vi "dcaccelerometer.vi"   [LabVIEW 2016]
uses:
  Scratch/FPGADCAccelerometer/DataTypes/DCAccelerometerSettings.ctl
  <vilib>/rvi/Emulation/niFpgaGetClockAttributes.vi
  <vilib>/rvi/Emulation/niFpgaSctlEmulationGetInTimedLoop.vi
  <vilib>/rvi/Emulation/niFpgaEmulationReportErrorSimple.vi
  <vilib>/rvi/Emulation/niFpgaEmulationIsFPGAContextNoSignature.vi
  <vilib>/rvi/errors/niFpgaSetErrorForExecOnDevCompSimple.vi
  <vilib>/rvi/eio/common/nirviEmuReportErrorAndStop.vi
  <vilib>/rvi/DataTransferAndStorage/Container/Common/niFpgaContainerGetUniqueNameForEmu.vi
  <vilib>/rvi/FIFO/Fifo_Resource/nirvififoEmulationSetSize.vi
  <vilib>/rvi/FIFO/Fifo_Resource/nirviFifoEmulationQueueMgr.vi
  <instcachedir>/0/nirviFifoEmulationQueueMgr_E5CAEC123FF24DC58D834DCA3CDAA9B5.lvgen/nirviFifoEmulationQueueMgr_E5CAEC123FF24DC58D834DCA3CDAA9B5_006.vi
  <vilib>/Utility/error.llb/Clear Errors.vi
  <vilib>/rvi/FIFO/Fifo_Resource/nirvififoEmulationCreateLock.vi
  <vilib>/rvi/Emulation/niFpgaProcessEmulError.vi
  <vilib>/rvi/FIFO/Fifo_Resource/nirvififoEmulationObtainLock.vi
  <vilib>/rvi/FIFO/Fifo_Resource/nirvififoEmulationReleaseLock.vi
  <vilib>/rvi/occurrence/nirviWaitOnOccurrenceBase.vi
  <vilib>/rvi/errors/nirviReportUnexpectedCaseInternalError.vi
  <vilib>/rvi/errors/nirviReportUnexpectedCaseInternalError (U32).vi
  <instcachedir>/0/nirviFifoEmulationQueueMgr_E5CAEC123FF24DC58D834DCA3CDAA9B5.lvgen/nirviFifoEmulationQueueMgr_E5CAEC123FF24DC58D834DCA3CDAA9B5_007.vi
  <vilib>/rvi/Emulation/niFpgaCriticalErrorInLSC.vi
  <vilib>/rvi/DataTransferAndStorage/Container/XNode/niFpgaContainer.xnode
  <vilib>/rvi/FIFO/Fifo_Resource/nirvififoEmulationRead.vi
  Scratch/FPGADCAccelerometer/FPGADCAccelerometer.lvlib
types:
  T1 = typedef "FPGADCAccelerometer.lvlib/DCAccelerometerSettings.ctl" = cluster{"AccelerometerClock":refnum<k21>, "AccelerometerX":refnum<k21>, "AccelerometerY":refnum<k21>, "AccelerometerZ":refnum<k21>, "TimestampRegister":refnum<k21>, "AccelerometerXDataFIFO":refnum<k21>, "AccelerometerYDataFIFO":refnum<k21>, "AccelerometerZDataFIFO":refnum<k21>, "AccelerometerTimestampFIFO":refnum<k21>}
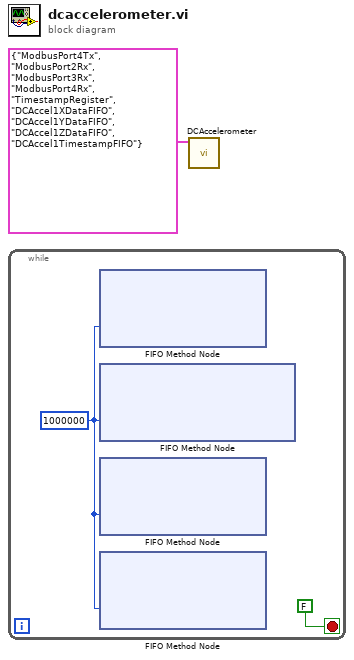
[diagram p0: block diagram]
diagram:
  n1 = while {
    stop <- FALSE stop-if-true
    w2 = 1000000 ("Timeout")
    n2 = xnode ("FIFO Method Node")("Timeout"=w2) -> ()  [unwired: 1 in, 3 out]
    n3 = xnode ("FIFO Method Node")("Timeout"=w2) -> ()  [unwired: 1 in, 3 out]
    n4 = xnode ("FIFO Method Node")("Timeout"=w2) -> ()  [unwired: 1 in, 3 out]
    n5 = xnode ("FIFO Method Node")("Timeout"=w2) -> ()  [unwired: 1 in, 3 out]
  }
  n6 = call "DCAccelerometer.vi"("DCAccelerometerSettings"=T1 {"AccelerometerClock"="ModbusPort4Tx", "AccelerometerX"="ModbusPort2Rx", "AccelerometerY"="ModbusPort3Rx", "AccelerometerZ"="ModbusPort4Rx", "TimestampRegister"="TimestampRegister", "AccelerometerXDataFIFO"="DCAccel1XDataFIFO", "AccelerometerYDataFIFO"="DCAccel1YDataFIFO", "AccelerometerZDataFIFO"="DCAccel1ZDataFIFO", "AccelerometerTimestampFIFO"="DCAccel1TimestampFIFO"}) -> ()  [unwired: 11 in]
